vi "3D-SegmentNameSection.vi"(0 "All Pos Data":string[][](array[string]), 5 "SegmentName":string) -> (4 "Selection Segment Pos":string[][](array[string]), 6 "X_StartPos":dbl, 8 "Y_StartPos":dbl, 10 "X_EndPos":dbl, 15 "Y_EndPos":dbl)   [LabVIEW 2015]
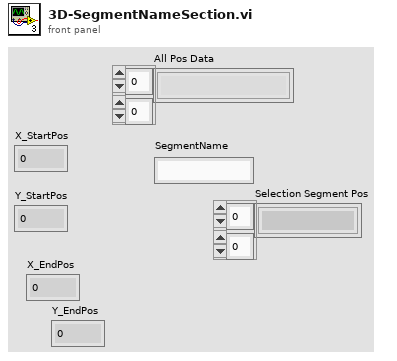
[diagram p1: front panel]
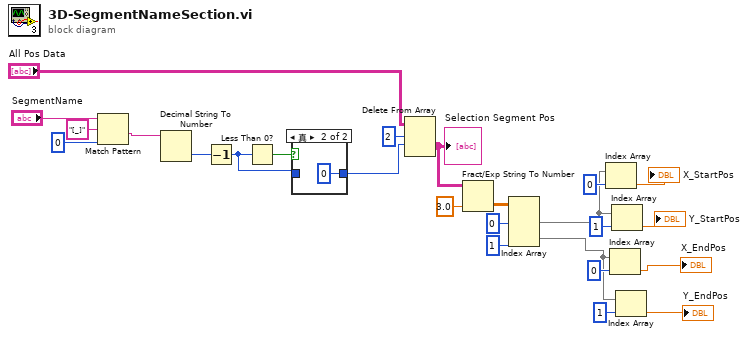
[diagram p0: block diagram]
diagram:
  n1 = Match Pattern(string="SegmentName", regular expression="[_]" ("正则表达式"), offset (0)=0 ("偏移量(0)")) -> (after substring=w22:string)  [unwired: 3 out]
  n2 = Decimal String To Number(string=w22) -> (number=w21:i32)  [unwired: 2 in, 1 out]
  n3 = Decrement(x=w21) -> (x-1=w17:i32)
  n4 = Less Than 0?(x=w17) -> (x < 0?=w18:bool)
  n5 = case shown="真" w18 {
    tunnel: w17 -> [w26 _]
    tunnel: [w26 0] -> w16
    frame False {
    }
    frame True {
    }
  }
  n6 = Delete From Array(array="All Pos Data", length=2 ("长度"), index (row)=w16) -> (deleted portion=w15:string[][])  [unwired: 1 in, 1 out]
  "Selection Segment Pos" <- w15
  n7 = Fract/Exp String To Number(string=w15, default (0 dbl)=3.0 ("默认(0 DBL)")) -> (number=w13:dbl[][])  [unwired: 2 in, 1 out]
  n8 = Index Array(array=w13, index (row) #1=0 ("索引 (行)"), index (col) #2=1 ("禁用的索引 (列)")) -> (element #1=w9:dbl[], element #2=w3:dbl[])  [unwired: 2 in]
  n9 = Index Array(array=w9, index=0 ("索引")) -> (element=→"X_StartPos":dbl)
  n10 = Index Array(array=w3, index=0 ("索引")) -> (element=→"X_EndPos":dbl)
  n11 = Index Array(array=w9, index=1 ("索引")) -> (element=→"Y_StartPos":dbl)
  n12 = Index Array(array=w3, index=1 ("索引")) -> (element=→"Y_EndPos":dbl)
